vi "Example_Host SPI Dual Port.vi"(0 "Port":i8, 1 "Configuration Cluster":T1={"CS"=1, "Clock Rate (Hz)"=50000.0, "Clock Mode"=2, "CS Active State"=FALSE} {"CS" items=["0"=1, "1"=2, "2"=4, "3"=8, "4"=16, "5"=32, "6"=64, "7"=128]; "Clock Mode" items=["0", "1", "2", "3"]}, 4 "Write Data":u8[](array[numeric]) format="%08b", 6 "Total Bits":u16=24, 9 "Hardware Pins":cluster{"RESET":bool, "LDAC":bool, "CLR":bool}={"RESET"=TRUE, "LDAC"=FALSE, "CLR"=TRUE}, 12 "Write":bool, 19 "stop":bool) -> (20 "Read Data":u8[](array[numeric]) format="%08b", 27 "error out":errorcluster)   [LabVIEW 2014]
uses:
  Host API/Controls/SPI Configuration Cluster.ctl
  <vilib>/FPGAPlugInAG/PXI-7852R/niLvFpga_Open_PXI-7852R.vi
  <vilib>/Utility/error.llb/Error Cluster From Error Code.vi
  <vilib>/RVI Host/nirviSupport.llb/nirviErrorClusterFromErrorCode.vi
  <vilib>/rvi/errors/niLvFpgaAdjustHostInterfaceError.vi
  <vilib>/FPGAPlugInAG/PXI-7852R/niLvFpga_Close_PXI-7852R.vi
  <vilib>/rvi/interface/nirviOpenFPGA/nirviOpenFPGA.xnode
  Host API/Controls/FPGA Reference.ctl
  FPGA Bitfiles/SPIExample_FPGATarget3_FPGASPIFPGATopLe_SKx8rjJlgp0.lvbitx
  FPGA/FPGA SPI_FPGA Top Level.vi
  <vilib>/rvi/interface/nirviMethod/nirviMethod.xnode
  <vilib>/rvi/interface/nirviCloseFPGA/nirviCloseFPGA.xnode
  <vilib>/rvi/interface/nirviMethod/StockFPGA_InlinedMethodWaitForSingleIRQ.vi
  <vilib>/FPGAPlugInAG/PXI-7852R/niLvFpga_WaitOnIrq_PXI-7852R.vi
  <vilib>/FPGAPlugInAG/PXI-7852R/niLvFpga_AcknowledgeIrq_PXI-7852R.vi
panel:
  in  "AD5781 Standard cmds":u16(ring) items=["Init DAC", "W DAC", "W CLR", "W Software CTRL", "R CLR"]
  # "Configure SPI"
  # "Write SPI"
  # "Control and Status"
  # "Read SPI"
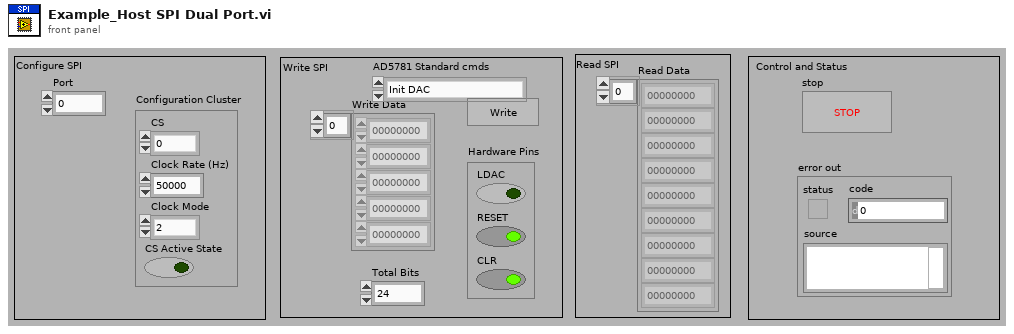
[diagram p1: front panel]
types:
  T1 = typedef "SPI Configuration Cluster.ctl" = cluster{"CS":u8, "Clock Rate (Hz)":dbl, "Clock Mode":u8, "CS Active State":bool}
  T2 = typedef "FPGA Reference.ctl" = refnum<k20>
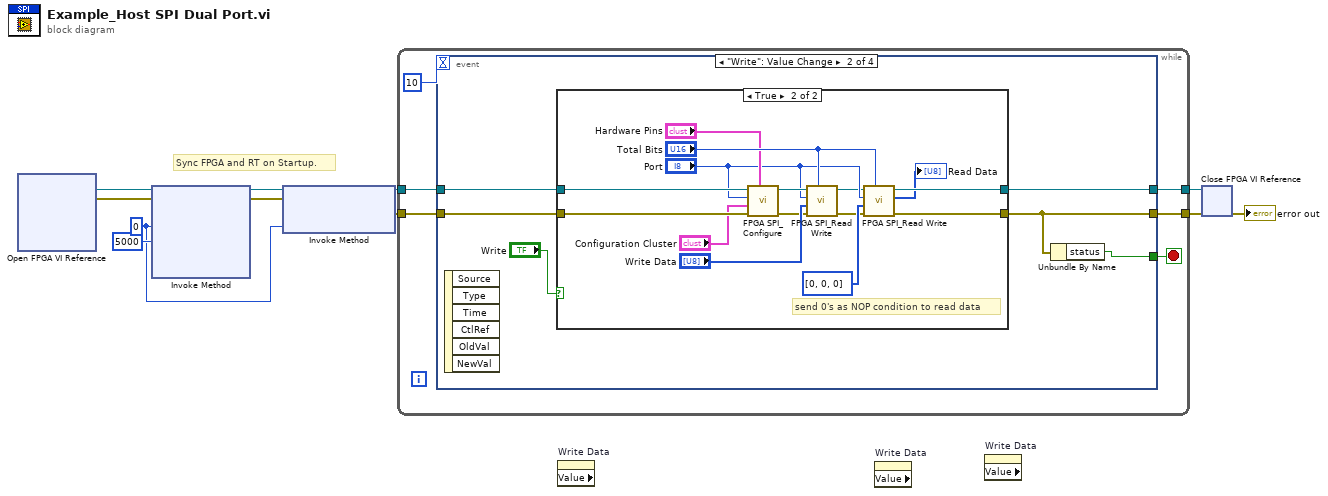
[diagram p0: block diagram]
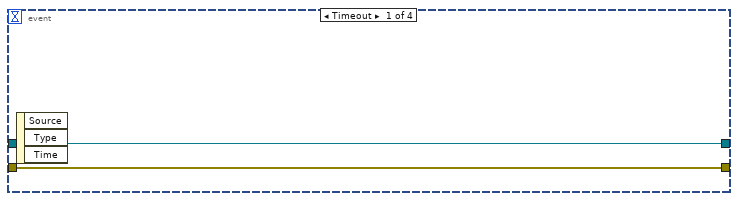
[diagram p2: hidden frame]
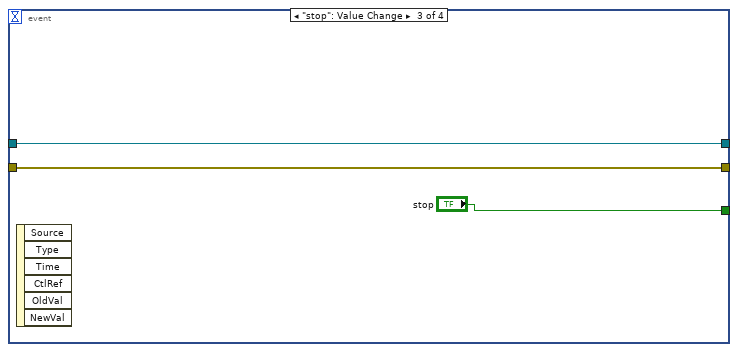
[diagram p4: hidden frame]
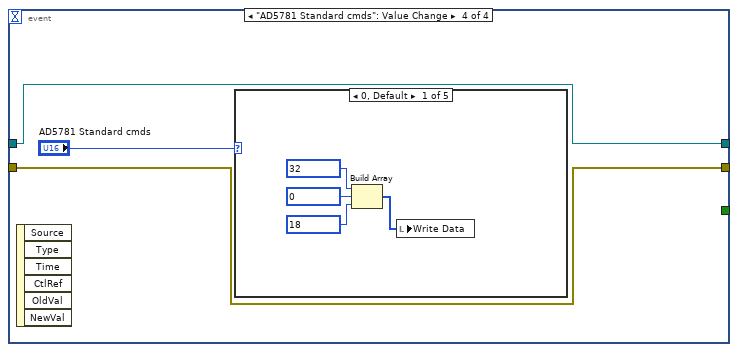
[diagram p5: hidden frame]
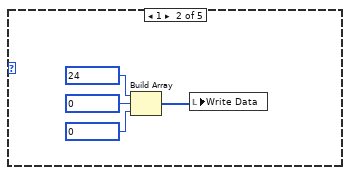
[diagram p6: hidden frame]
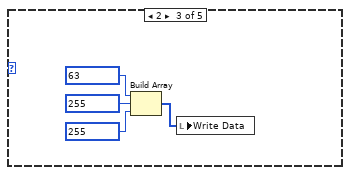
[diagram p7: hidden frame]
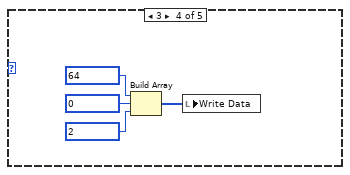
[diagram p8: hidden frame]
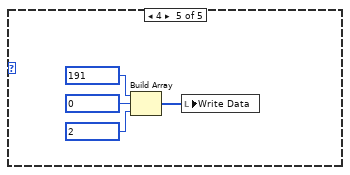
[diagram p9: hidden frame]
diagram:
  w1 = 0 ("IRQ Number(s)")
  # "Sync FPGA and RT on Startup."
  n1 = xnode "Open FPGA VI Reference"() -> ("FPGA VI Reference Out"=w8:T2, "error out"=w7:errorcluster)  [unwired: 2 in]
  n2 = xnode "Invoke Method"("FPGA VI Reference In"=w8, "error in"=w7, "IRQ Number(s)"=w1, "Timeout (ms)"=5000) -> ("FPGA VI Reference Out"=w6:T2, "error out"=w5:errorcluster)  [unwired: 2 out]
  n3 = xnode "Invoke Method"("FPGA VI Reference In"=w6, "error in"=w5, "IRQ Number(s)"=w1) -> ("FPGA VI Reference Out"=w3:T2, "error out"=w2:errorcluster)
  n4 = while {
    tunnel: w3 -> [w17]
    tunnel: w2 -> [w16]
    tunnel: [w15] -> w11
    tunnel: [w14] -> w10
    stop <- w12 stop-if-true
    n5 = event shown="[1] \"Write\": Value Change" {
      selector: _ -> [_ _ _ _]
      dyn-events: _ -> [_ _ _ _]
      timeout: 10 ("Count(mSec)") -> [_ _ _ _]
      tunnel: w17 -> [w19 w25 w44 w47]
      tunnel: w16 -> [w18 w24 w43 w46]
      tunnel: [w19 w23 w44 w47] -> w15
      tunnel: [w18 w22 w43 w46] -> w14
      tunnel: [_ w21 "stop" _] -> w12
      event Timeout {
        n6 = event-data() -> ()  [unwired: 1 in, 3 out]
      }
      event "Write": Value Change {
        n7 = event-data() -> ()  [unwired: 1 in, 6 out]
        n8 = case shown="True" "Write" {
          tunnel: w25 -> [w27 w42]
          tunnel: w24 -> [w26 w41]
          tunnel: [w27 w34] -> w23
          tunnel: [w26 w35] -> w22
          frame False {
          }
          frame True {
            # "send 0's as NOP condition to read data"
            n9 = call "FPGA SPI_Configure.vi"("Hardware Pins"="Hardware Pins", "error in"=w41, "Configuration Cluster"="Configuration Cluster", "Port"="Port", "FPGA Interface"=w42) -> ("error out"=w38:errorcluster, "FPGA VI Reference Out"=w39:refnum<k20>)  [unwired: 5 out]
            n10 = call "FPGA SPI_Read Write.vi"("Total Bits"="Total Bits", "error in"=w38, "Write Data"="Write Data", "Port"="Port", "FPGA Interface"=w39) -> ("error out"=w28:errorcluster, "FPGA VI Reference Out"=w29:refnum<k20>)  [unwired: 5 out]
            n11 = call "FPGA SPI_Read Write.vi"("Total Bits"="Total Bits", "error in"=w28, "Write Data"=u8[] [0, 0, 0], "Port"="Port", "FPGA Interface"=w29) -> ("error out"=w35:errorcluster, "Read Data"=→"Read Data":u8[], "FPGA VI Reference Out"=w34:refnum<k20>)  [unwired: 4 out]
          }
        }
        n12 = Unbundle By Name(w22) -> ("status"=w21:bool)
      }
      event "stop": Value Change {
        n13 = event-data() -> ()  [unwired: 1 in, 6 out]
      }
      event "AD5781 Standard cmds": Value Change {
        n14 = event-data() -> ()  [unwired: 1 in, 6 out]
        n15 = case shown="0, Default" "AD5781 Standard cmds" {
          frame 0, Default {
            n16 = Build Array(u8 32, u8 0, u8 18) -> (w49:u8[])
            n17 = local write "Write Data"(w49) -> ()
          }
          frame 1 {
            n18 = Build Array(u8 24, u8 0, u8 0) -> (w53:u8[])
            n19 = local write "Write Data"(w53) -> ()
          }
          frame 2 {
            n20 = Build Array(u8 63, u8 255, u8 255) -> (w57:u8[])
            n21 = local write "Write Data"(w57) -> ()
          }
          frame 3 {
            n22 = Build Array(u8 64, u8 0, u8 2) -> (w61:u8[])
            n23 = local write "Write Data"(w61) -> ()
          }
          frame 4 {
            n24 = Build Array(u8 191, u8 0, u8 2) -> (w65:u8[])
            n25 = local write "Write Data"(w65) -> ()
          }
        }
      }
    }
  }
  n26 = property on="Write Data" class="Arr (strict)" props=["Value"]() -> ()  [unwired: 2 in, 3 out]
  n27 = property on="Write Data" class="Arr (strict)" props=["Value"]() -> ()  [unwired: 2 in, 3 out]
  n28 = property on="Write Data" class="Arr (strict)" props=["Value"]() -> ()  [unwired: 2 in, 3 out]
  n29 = xnode "Close FPGA VI Reference"("FPGA VI Reference In"=w11, "error in"=w10) -> ("error out"=→"error out":errorcluster)
